vi "Practica-for-shift-y-arreglos.vi"() -> ()   [LabVIEW 2018]
panel:
  out "Prueba":dbl[](array[numeric])
  out "Menor a mayor":dbl[](array[numeric])
  out "Valor minimo":dbl
  out "Valor maximo":dbl
  out "Array":dbl[](array[numeric])
  out "Numeric 2":dbl
  out "Numeric":dbl
  out "Waveform Chart":dbl(graph)
  in  "stop":bool
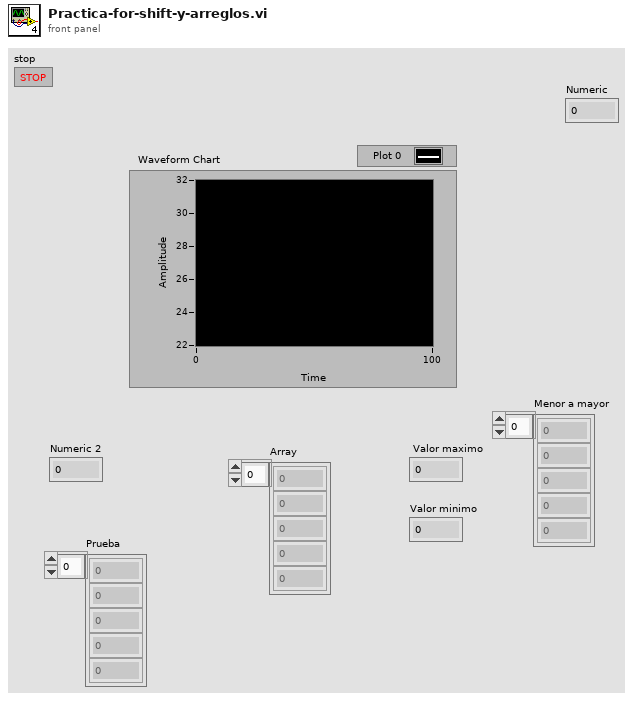
[diagram p1: front panel]
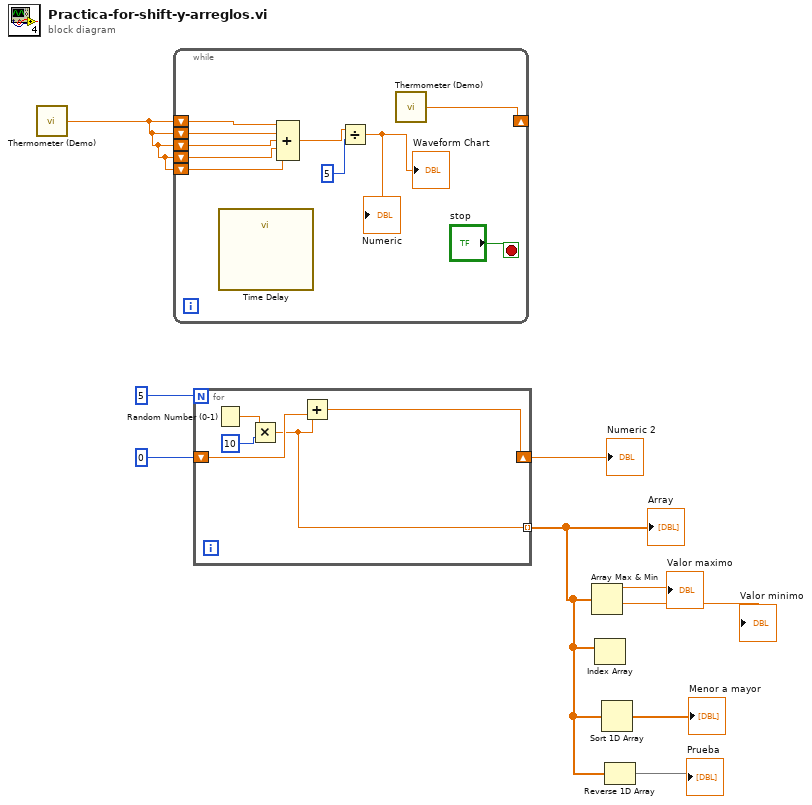
[diagram p0: block diagram]
diagram:
  n1 = call "Thermometer (Demo).vi"() -> ("Temperature Value"=w9:dbl)  [unwired: 1 in]
  n2 = while {
    shift-right: [w11] -> _
    shift-left: w9 -> [w18]
    shift-left: w9 -> [w17]
    shift-left: w9 -> [w16]
    shift-left: w9 -> [w15]
    shift-left: w9 -> [w14]
    stop <- "stop" stop-if-true
    n3 = call "Time Delay"() -> ()  [unwired: 11 in, 1 out]
    n4 = Compound Arithmetic op=ADD(w18, w17, w16, w15, w14) -> (w13:dbl)
    n5 = Divide(x=w13, y=5) -> (x/y=→"Waveform Chart" →"Numeric":dbl)
    n6 = call "Thermometer (Demo).vi"() -> ("Temperature Value"=w11:dbl)  [unwired: 1 in]
  }
  n7 = for {
    N: 5 -> [_]
    shift-right: [w23] -> w6
    shift-left: 0 -> [w24]
    tunnel: [w20] -> w2 mode=indexing
    n8 = Random Number (0-1)() -> (number: 0 to 1=w22:dbl)
    n9 = Multiply(x=w22, y=10) -> (x*y=w20:dbl)
    n10 = Add(x=w20, y=w24) -> (x+y=w23:dbl)
  }
  "Numeric 2" <- w6
  "Array" <- w2
  n11 = Array Max & Min(array=w2) -> (max value=→"Valor maximo":dbl, min value=→"Valor minimo":dbl)  [unwired: 2 out]
  n12 = Index Array(array=w2) -> ()  [unwired: 1 in, 1 out]
  n13 = Sort 1D Array(array=w2) -> (sorted array=→"Menor a mayor":dbl[])
  n14 = Reverse 1D Array(array=w2) -> (reversed array=→"Prueba":dbl[])
